vi "GetCursorPos.vi"() -> (3 "cursor position":cluster{"x":i16, "y":i16})   [LabVIEW 2011]
doc: "GetCursorPos\nThe GetCursorPos function retrieves the cursor's position, in screen coordinates. \n\nBOOL GetCursorPos(\n LPPOINT lpPoint // address of structure for cursor position\n);\n \nParameters\nlpPoint \nPointer to aPOINT structure that receives the screen coordinates of the cursor. \nReturn Values\nIf the function succeeds, the return value is nonzero.\n\nIf the function fails, the return value is zero. To get extended error information, callGetLastError.\n\nRemarks\nThe cursor position is always given in screen coordinates and is not affected by the mapping mode of the window that contains the cursor. \n\nThe calling process must have WINSTA_READATTRIBUTES access to the window station."
uses:
  user32.dll
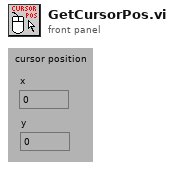
[diagram p1: front panel]
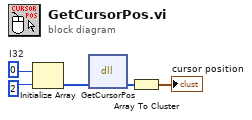
[diagram p0: block diagram]
diagram:
  w5 = 0  # I32
  n1 = Initialize Array(w5, 2) -> (w3:i32[])
  n2 = dll-call lib="User32.dll" fn="GetCursorPos"("POINT"=w3) -> ("POINT"=w2:i32[])  [unwired: 3 in, 3 out]
  n3 = Array To Cluster(array=w2) -> (cluster=→"cursor position":cluster{"POINT[0]":i32, "POINT[1]":i32})
